vi "ProduceGraphFromDropletDbs.vi"(8 "error in (no error)":errorcluster, 11 "Droplets Freeze Information":T1) -> (0 "error out":errorcluster, 1 "Median":dbl, 2 "NoOfDroplets":i32, 3 "Normalized number of Droplets vs. Temperature":cluster{"Ramp Pattern":dbl[], dbl[]}(graph))   [LabVIEW 2013]
doc: "Use this template to build a VI to use as a subVI."
uses:
  TypeDef/MultipleFileData.ctl
  <vilib>/Analysis/1siggen.llb/Ramp Pattern by Delta.vi
  <vilib>/Analysis/NI_AALBase.lvlib
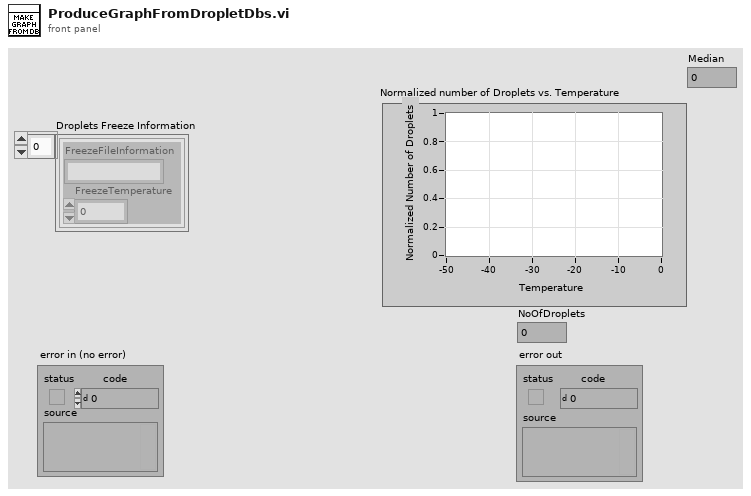
[diagram p1: front panel]
types:
  T1 = typedef "MultipleFileData.ctl" = cluster{"FreezeTemperature":dbl, "FreezeFileInformation":string}[]
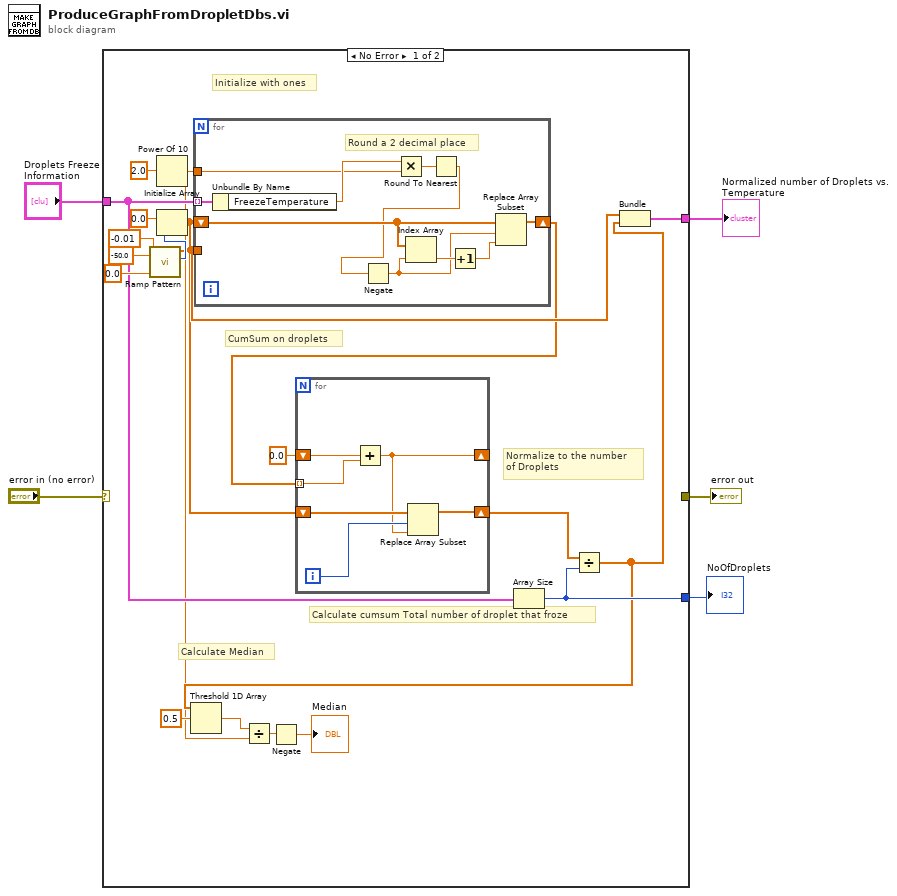
[diagram p0: block diagram]
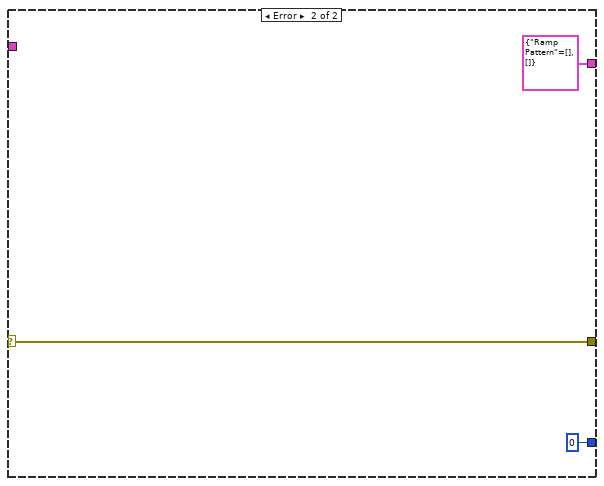
[diagram p2: hidden frame]
diagram:
  n1 = case shown="No Error" "error in (no error)" {
    selector: "error in (no error)" -> [_ w44]
    tunnel: [_ w44] -> w4
    tunnel: "Droplets Freeze Information" -> [w22 _]
    tunnel: [w18 cluster{"Ramp Pattern":dbl[], dbl[]} {"Ramp Pattern"=[], []}] -> w2
    tunnel: [w14 0] -> w1
    frame No Error {
      # "Calculate Median"
      # "Normalize to the number \nof Droplets"
      # "Calculate cumsum Total number of droplet that froze"
      # "CumSum on droplets"
      # "Initialize with ones"
      n2 = call-poly <vilib>:"Ramp Pattern.vi"("start"=0.0, "end"=-50.0, "delta"=-0.01) -> ("samples"=w21:i32, "Ramp Pattern"=w19:dbl[])  [unwired: 6 in, 1 out]
      n3 = Power Of 10(x=2.0) -> (10^x=w6:dbl)
      n4 = Initialize Array(0.0 ("element"), w21) -> (w16:dbl[])
      n5 = for {
        tunnel: w22 -> [w41] mode=indexing
        tunnel: w19 -> [_]
        shift-right: [w37] -> w13
        shift-left: w16 -> [w38]
        tunnel: w6 -> [w32]
        # "Round a 2 decimal place"
        n6 = Unbundle By Name(w41) -> ("FreezeTemperature"=w35:dbl)
        n7 = Multiply(x=w35, y=w32) -> (x*y=w36:dbl)
        n8 = Round To Nearest(number=w36) -> (nearest integer value=w34:dbl)
        n9 = Negate(x=w34) -> (-x=w33:dbl)
        n10 = Index Array(array=w38, index=w33) -> (element=w40:dbl)
        n11 = Increment(x=w40) -> (x+1=w39:dbl)
        n12 = Replace Array Subset(array=w38, new element=w39, index=w33) -> (w37:dbl[])
      }
      n13 = for {
        tunnel: w13 -> [w30] mode=indexing
        shift-right: [w26] -> w15
        shift-left: w16 -> [w29]
        shift-right: [w27] -> _
        shift-left: 0.0 -> [w31]
        i -> [w28]
        n14 = Add(x=w31, y=w30) -> (x+y=w27:dbl)
        n15 = Replace Array Subset(array=w29, new element=w27, index=w28) -> (w26:dbl[])
      }
      n16 = Array Size(array=w22) -> (size(s)=w14:i32)
      n17 = Divide(x=w15, y=w14) -> (x/y=w11:dbl[])
      n18 = Threshold 1D Array(2:0.5 ("threshold y"), 3:w11) -> (0:w9:dbl)  [unwired: 1 in]
      n19 = Divide(x=w9, y=w6) -> (x/y=w8:dbl)
      n20 = Negate(x=w8) -> (-x=→"Median":dbl)
      n21 = Bundle("Ramp Pattern"=w19, w11) -> (w18:cluster{"Ramp Pattern":dbl[], dbl[]})  [unwired: 1 in]
    }
    frame Error {
    }
  }
  "error out" <- w4
  "Normalized number of Droplets vs. Temperature" <- w2
  "NoOfDroplets" <- w1
